vi "testGetTargetIPAddressesMatchesSystemDefinition.vi"(8 "error in (no error)":errorcluster, 11 "TestCase in":refnum<class "VeriStandTestCaseUnitTests.lvclass">) -> (0 "error out":errorcluster, 3 "TestCase out":refnum<class "VeriStandTestCaseUnitTests.lvclass">)   [LabVIEW 2015, in "VeriStandTestCaseUnitTests.lvclass"]
uses:
  VeriStandTestCaseUnitTests.lvclass
  <vilib>/addons/_JKI Toolkits/VI Tester/TestCase.llb/TestCase.lvclass
  VeriStandTestCase.lvclass
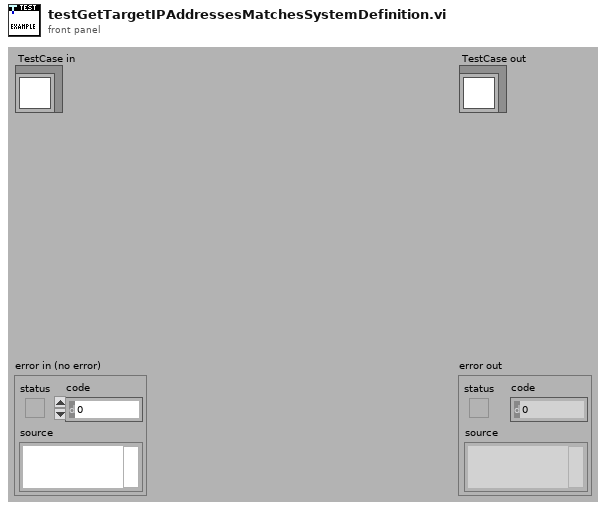
[diagram p1: front panel]
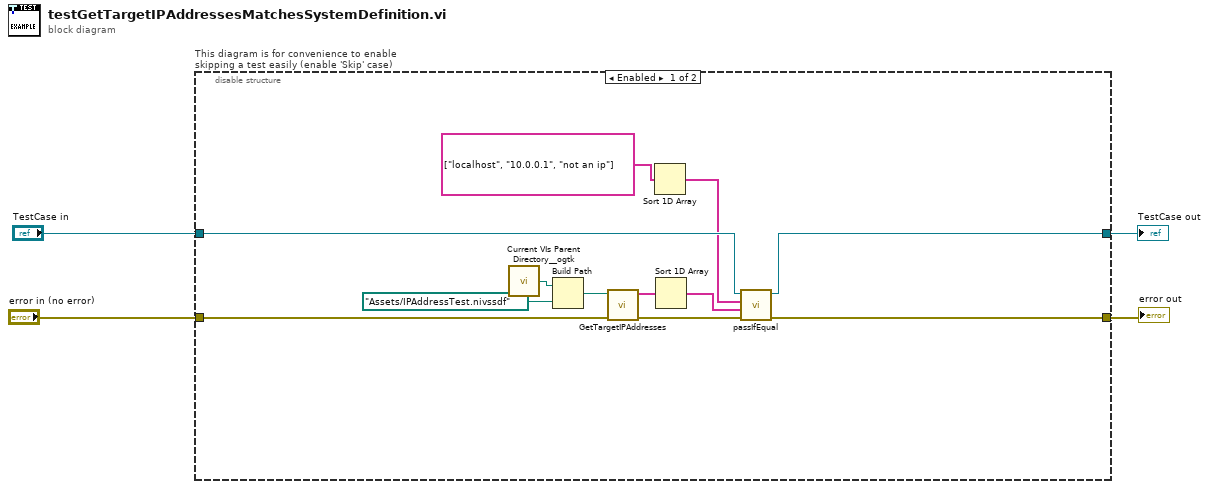
[diagram p0: block diagram]
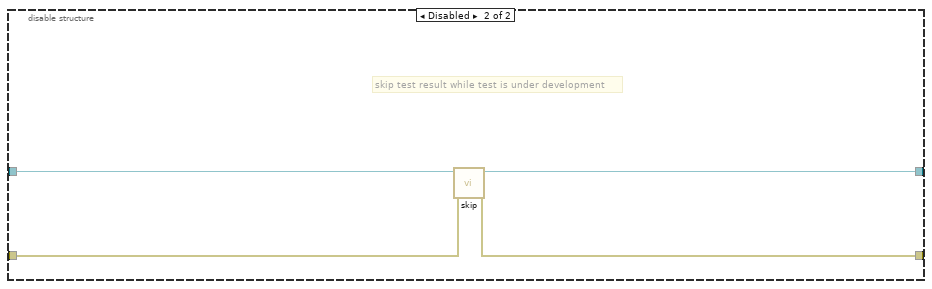
[diagram p2: hidden frame]
diagram:
  n1 = disable-structure "This diagram is for convenience to enable skipping a test easily (enable 'Skip' case)" shown="Enabled" {
    disable-tunnel: "TestCase in" -> [w7 w20]
    disable-tunnel: [w8 w18] -> w1
    disable-tunnel: [w9 w19] -> w3
    disable-tunnel: "error in (no error)" -> [w16 w17]
    frame Enabled {
      n2 = call <userlib>:"Current VIs Parent Directory__ogtk.vi"() -> ("Parent Directory (+ Relative)"=w15:path)  [unwired: 5 in]
      n3 = Build Path(base path=w15, name or relative path=path "Assets/IPAddressTest.nivssdf" ("absolute system definition file")) -> (appended path=w13:path)
      n4 = call "GetTargetIPAddresses.vi"("error in (no error)"=w16, "absolute system definition file"=w13) -> ("error out"=w10:errorcluster, "ip addresses"=w12:string[])  [unwired: 8 in]
      n5 = Sort 1D Array(array=string[] ["localhost", "10.0.0.1", "not an ip"] ("string array")) -> (sorted array=w5:string[])
      n6 = Sort 1D Array(array=w12) -> (sorted array=w11:string[])
      n7 = call-dynamic "passIfEqual.vi"("error in (no error)"=w10, "y"=w11, "x"=w5, "TestCase in"=w7) -> ("error out"=w9:errorcluster, "TestCase out"=w8:refnum<class "VeriStandTestCaseUnitTests.lvclass">)  [unwired: 6 in]
    }
    frame Disabled {
      # "skip test result while test is under development"
      n8 = call <vilib>:"skip.vi"("error in (no error)"=w17, "TestCase in"=w20) -> ("error out"=w19:errorcluster, "TestCase out"=w18:refnum<class "VeriStandTestCaseUnitTests.lvclass">)  [unwired: 8 in]
    }
  }
  "error out" <- w3
  "TestCase out" <- w1
